vi "Client State String.vi"(4 "S in":refnum<vi>, 5 "String":string, 6 "Sync":variant) -> (7 "S":refnum<vi>)   [LabVIEW 2020, in "Vecto.lvlib" / "TCPMessaging.lvclass"]
uses:
  TCPMessaging.lvclass
  TCPMessaging.lvclass/TCPMessaging.ctl
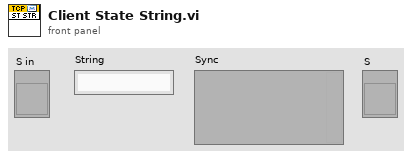
[diagram p1: front panel]
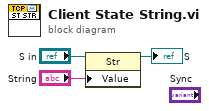
[diagram p0: block diagram]
diagram:
  n1 = property class="Str"(reference="S in", "Value"="String") -> (reference out=→"S":refnum<vi>)  [unwired: 1 in, 1 out]
